vi "FlatToRichtest_service_WaitRequest.vi"(5 "OutputClusterType":T1, 11 "InputCluster":T2) -> (3 "OutputCluster":T1)   [LabVIEW 2021, in "test_service_server.lvlib"]
uses:
  test_service_server.lvlib
  test_service_WaitRequest_Flat.ctl
  test_service_WaitRequest.ctl
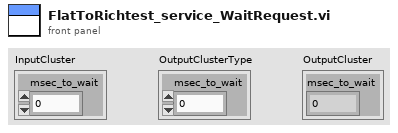
[diagram p1: front panel]
types:
  T1 = typedef "test_service_server.lvlib/test_service_WaitRequest.ctl" = cluster{"msec_to_wait":u64}
  T2 = typedef "test_service_server.lvlib/test_service_WaitRequest_Flat.ctl" = cluster{"msec_to_wait":u64}
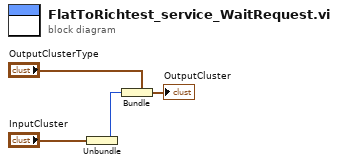
[diagram p0: block diagram]
diagram:
  n1 = Unbundle "Unbundle"("InputCluster") -> ("msec_to_wait"=w1:u64)
  n2 = Bundle "Bundle"(cluster="OutputClusterType", "msec_to_wait"=w1) -> (→"OutputCluster":T1)
